vi "Database_Init.vi"(8 "error in (no error)":errorcluster, 10 "path":path, 11 "object in":refnum<class "Database.lvclass">) -> (0 "error out":errorcluster, 3 "object out":refnum<class "Database.lvclass">)   [LabVIEW 2015, in "Database.lvclass"]
uses:
  Database.lvclass
  Database.lvclass/Database.ctl
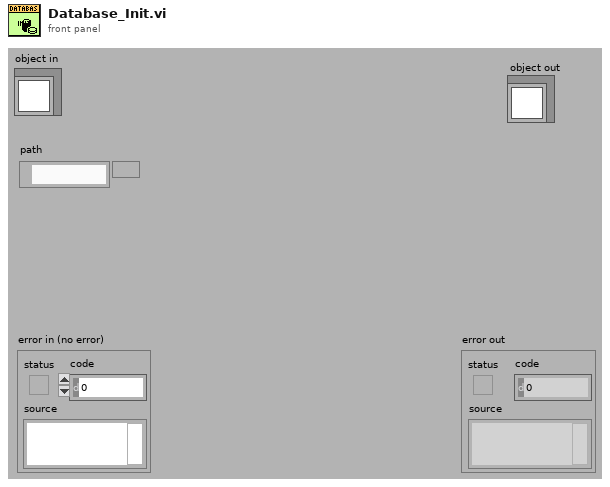
[diagram p1: front panel]
types:
  T1 = enum16{"open", "replace", "create", "open or create", "replace or create", "replace or create with confirmation"}
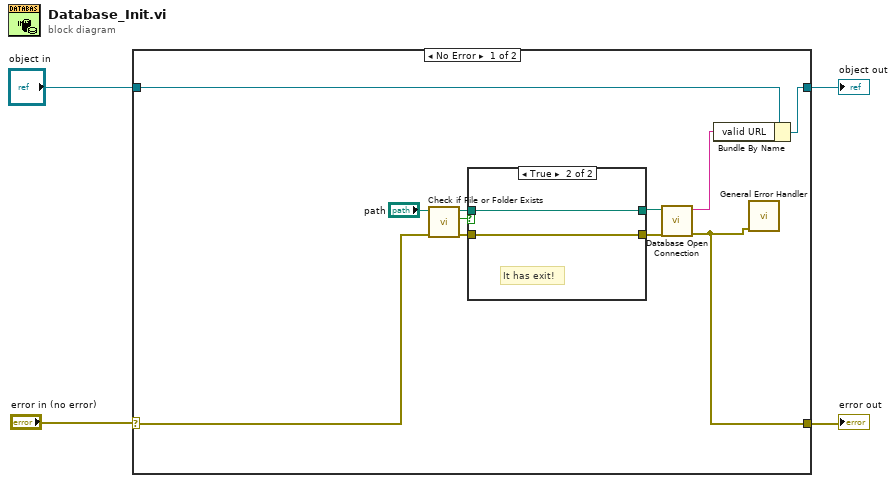
[diagram p0: block diagram]
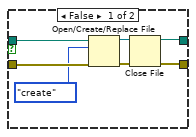
[diagram p2: hidden frame]
diagram:
  n1 = case shown="No Error" "error in (no error)" {
    selector: "error in (no error)" -> [w15 w25]
    tunnel: "object in" -> [w10 w26]
    tunnel: [w8 w26] -> w3
    tunnel: [w7 w25] -> w1
    frame No Error {
      n2 = call <vilib>:"Check if File or Folder Exists.vi"("error in (no error)"=w15, "path"="path") -> ("error out"=w12:errorcluster, "file or folder exists?"=w14:bool, "dup path"=w13:path)  [unwired: 7 in]
      n3 = case shown="True" w14 {
        tunnel: w13 -> [w22 w24]
        tunnel: w12 -> [w21 w23]
        tunnel: [w17 w24] -> w5
        tunnel: [w16 w23] -> w11
        frame False {
          n4 = Open/Create/Replace File(file path (use dialog)=w22, error in=w21, operation (0:open)=T1."create") -> (refnum out=w19:refnum<file>, error out=w18:errorcluster)  [unwired: 3 in, 1 out]
          n5 = Close File(refnum=w19, error in=w18) -> (path=w17:path, error out=w16:errorcluster)
        }
        frame True {
          # "It has exit!"
        }
      }
      n6 = call "Database Open Connection.vi"("error in"=w11, "File Path"=w5) -> ("error out"=w7:errorcluster, "valid URL"=w9:string)  [unwired: 8 in]
      n7 = Bundle By Name(cluster=w10, "valid URL"=w9) -> (w8:refnum<class "Database.lvclass">)
      n8 = call <vilib>:"General Error Handler.vi"("error in (no error)"=w7) -> ()  [unwired: 10 in, 5 out]
    }
    frame Error {
    }
  }
  "object out" <- w3
  "error out" <- w1
